vi "Decrypt_Selected_File_of_Hierarchy_Data_inside.vi"(8 "error in (no error)":errorcluster, 9 "FileName":string, 10 "SubFolderName":string, 11 "object in":refnum<class "Crypter.lvclass">) -> (0 "error out":errorcluster, 1 "Folder_Mgmt out":refnum<class "Folder_Mgmt.lvclass">, 2 "Dencrypted text":string, 3 "object out":refnum<class "Crypter.lvclass">)   [LabVIEW 2016, in "Crypter.lvclass"]
uses:
  Crypter.lvclass
  C:/Users/Marco Preziani/Documents/DOME-LV16/WebBrowser_Mgmt/WebBrowser_Mgmt.lvclass
  Folder_Mgmt/Folder_Mgmt.lvclass
  WebBrowser_Mgmt/WebBrowser_Mgmt.lvclass/WebBrowser_Mgmt.ctl
  Folder_Mgmt/Folder_Mgmt.lvclass/Folder_Mgmt.ctl
  WebBrowser_Mgmt/WebBrowser_Mgmt.lvclass
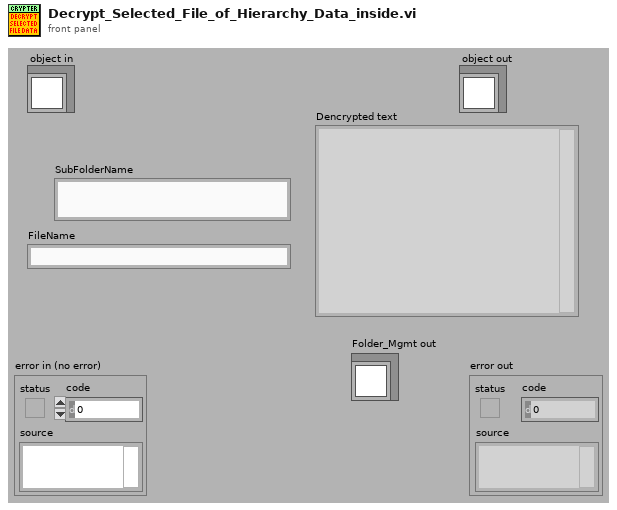
[diagram p1: front panel]
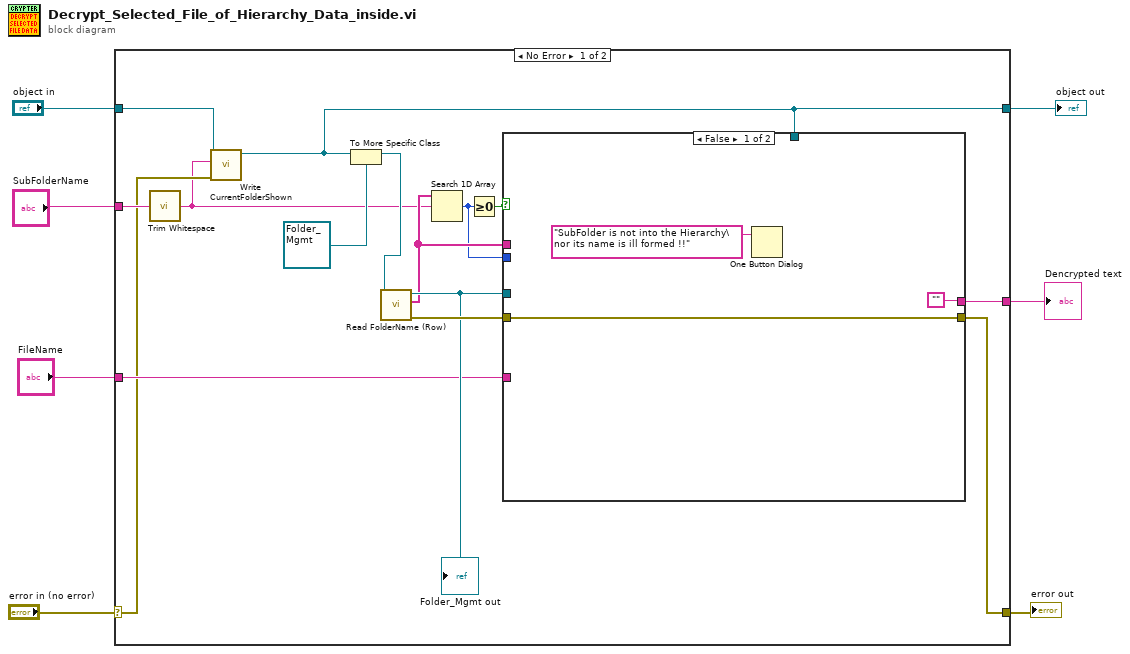
[diagram p0: block diagram]
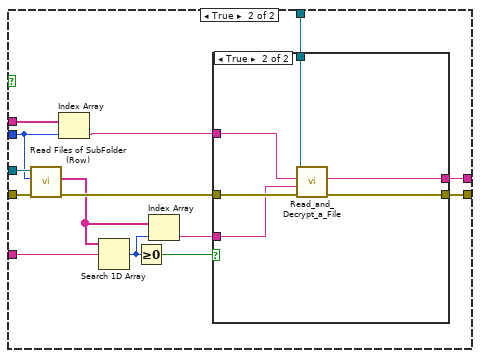
[diagram p2: hidden frame]
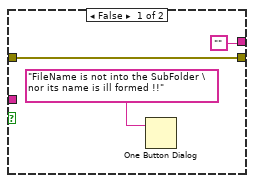
[diagram p3: hidden frame]
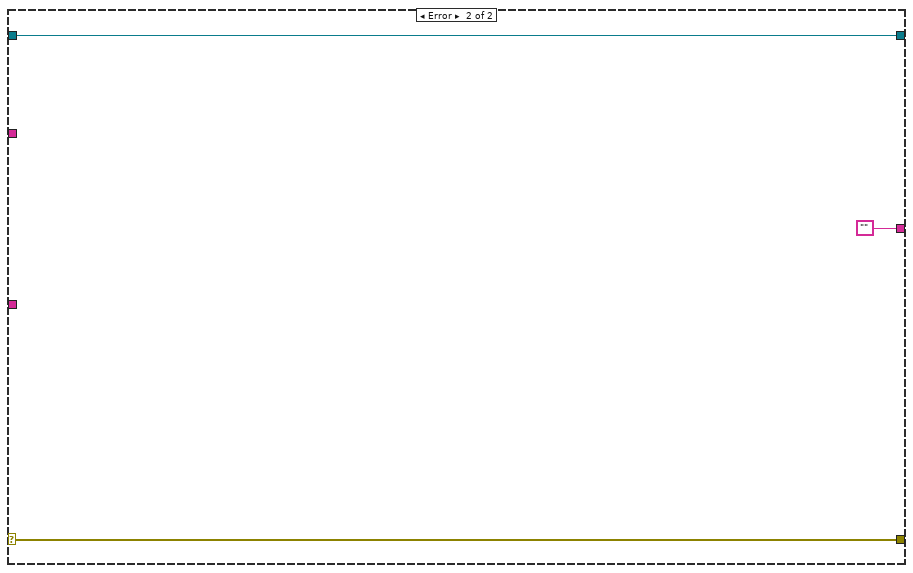
[diagram p4: hidden frame]
diagram:
  n1 = case shown="No Error" "error in (no error)" {
    selector: "error in (no error)" -> [w13 w51]
    tunnel: [w22 w51] -> w6
    tunnel: [w8 w50] -> w4
    tunnel: "object in" -> [w12 w50]
    tunnel: "SubFolderName" -> [w20 _]
    tunnel: "FileName" -> [w15 _]
    tunnel: [w14 ""] -> w1
    frame No Error {
      n2 = call <vilib>:"Trim Whitespace.vi"("string"=w20) -> ("trimmed string"=w9:string)  [unwired: 1 in]
      n3 = call "Write CurrentFolderShown.vi"("error in (no error)"=w13, "CurrentFolderShown"=w9, "WebBrowser_Mgmt in"=w12) -> ("WebBrowser_Mgmt out"=w8:refnum<class "Crypter.lvclass">)  [unwired: 7 in, 1 out]
      n4 = To More Specific Class(target class=refnum<class "Folder_Mgmt.lvclass"> refnum ("Folder_Mgmt.lvclass"), reference=w8) -> (specific class reference=w10:refnum<class "Folder_Mgmt.lvclass">)  [unwired: 1 in, 1 out]
      n5 = call "Read FolderName (Row).vi"("Folder_Mgmt in"=w10) -> ("error out"=w21:errorcluster, "FolderName (Row)"=w18:string[], "Folder_Mgmt out"=w19:refnum<class "Folder_Mgmt.lvclass">)  [unwired: 8 in]
      "Folder_Mgmt out" <- w19
      n6 = Search 1D Array(1D array=w18, element=w9) -> (index of element=w17:i32)  [unwired: 1 in]
      n7 = Greater Or Equal To 0?(x=w17) -> (x >= 0?=w16:bool)
      n8 = case shown="False" w16 {
        tunnel: [w25 w30] -> w22
        tunnel: w21 -> [w25 w39]
        tunnel: w19 -> [_ w38]
        tunnel: w18 -> [_ w36]
        tunnel: w17 -> [_ w29]
        tunnel: w15 -> [_ w34]
        tunnel: ["" w27] -> w14
        tunnel: w8 -> [_ w26]
        frame False {
          n9 = One Button Dialog(message="SubFolder is not into the Hierarchy\nor its name is ill formed !!") -> ()  [unwired: 1 in, 1 out]
        }
        frame True {
          n10 = call "Read Files of SubFolder (Row).vi"("error in (no error)"=w39, "RowIndex"=w29, "Folder_Mgmt in"=w38) -> ("error out"=w37:errorcluster, "FolderFiles (Row)"=w32:string[])  [unwired: 6 in, 1 out]
          n11 = Index Array(array=w36, index=w29) -> (element=w35:string)
          n12 = Search 1D Array(1D array=w32, element=w34) -> (index of element=w33:i32)  [unwired: 1 in]
          n13 = Greater Or Equal To 0?(x=w33) -> (x >= 0?=w28:bool)
          n14 = Index Array(array=w32, index=w33) -> (element=w31:string)
          n15 = case shown="True" w28 {
            tunnel: w37 -> [w41 w48]
            tunnel: w35 -> [_ w47]
            tunnel: w31 -> [_ w46]
            tunnel: [w41 w45] -> w30
            tunnel: ["" w44] -> w27
            tunnel: w26 -> [_ w43]
            frame False {
              n16 = One Button Dialog(message="FileName is not into the SubFolder \nor its name is ill formed !!") -> ()  [unwired: 1 in, 1 out]
            }
            frame True {
              n17 = call-dynamic "Read_and_Decrypt_a_File.vi"("error in (no error)"=w48, "name of File"=w46, "name of Folder"=w47, "object in"=w43) -> ("error out"=w45:errorcluster, "Dencrypted text"=w44:string)  [unwired: 5 in, 1 out]
            }
          }
        }
      }
    }
    frame Error {
    }
  }
  "error out" <- w6
  "object out" <- w4
  "Dencrypted text" <- w1
